vi "Array Metadata.vi"(8 "error in (no error)":errorcluster, 11 "Array":variant) -> (0 "error out":errorcluster, 2 "number of dimensions":u32, 3 "Value":string)   [LabVIEW 2019, in "BlueVariantView.lvlib"]
uses:
  BlueVariantView.lvlib
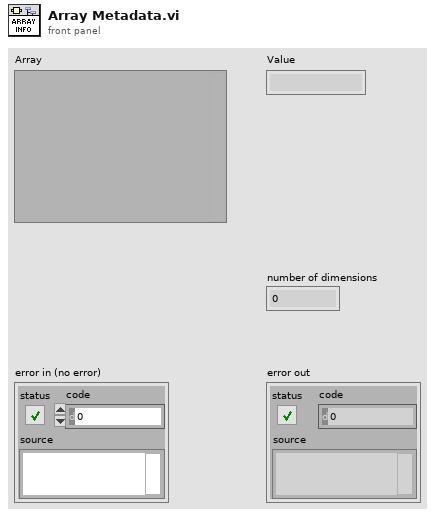
[diagram p1: front panel]
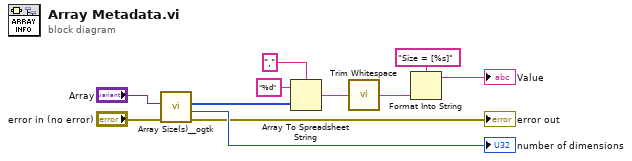
[diagram p0: block diagram]
diagram:
  n1 = call <userlib>:"Array Size(s)__ogtk.vi"("error in (no error)"="error in (no error)", "Array"="Array") -> ("error out"=→"error out":errorcluster, "N dims"=→"number of dimensions":u32, "Size(s)"=w4:u32[])  [unwired: 7 in]
  n2 = Array To Spreadsheet String(delimiter (Tab)=",", array=w4, 3:"%d" ("format string")) -> (spreadsheet string=w8:string)
  n3 = call <vilib>:"Trim Whitespace.vi"("string"=w8) -> ("trimmed string"=w7:string)  [unwired: 1 in]
  n4 = Format Into String(format string="Size = [%s]", w7) -> (resulting string=→"Value":string)  [unwired: 2 in, 1 out]
